vi "Combine Error.vi"(1 "Error #4":errorcluster, 2 "Error #3":errorcluster, 3 "Error #2":errorcluster, 4 "Error #1":errorcluster) -> (0 "Error Out":errorcluster)   [LabVIEW 2020]
doc: "Combines multiple error cluster into a single error cluster. If any of the inputs have an error, then Error Out will reflect the first error. If none of the inputs have errors, error out will show no error."
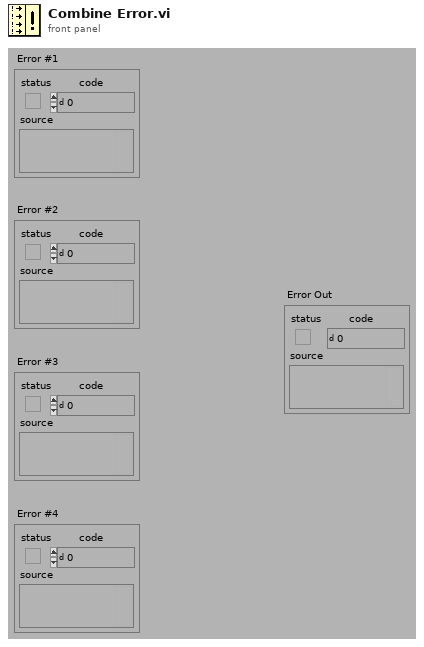
[diagram p1: front panel]
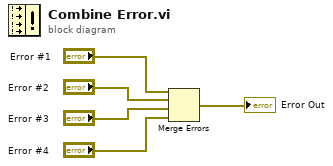
[diagram p0: block diagram]
diagram:
  n1 = Merge Errors("Error #1", "Error #2", "Error #3", "Error #4") -> (→"Error Out":errorcluster)
